vi "getRelPositions.vi"(9 "originOffsetVectors":T2, 10 "point":T1, 11 "mountOn":enum16{"yArm", "breadBoard"}(ring)) -> (2 "to_yPOI":T1, 3 "to_BBorigin":T1)   [LabVIEW 2015]
uses:
  <vilib>/Utility/miscctls.llb/LV3DPointTypeDef.ctl
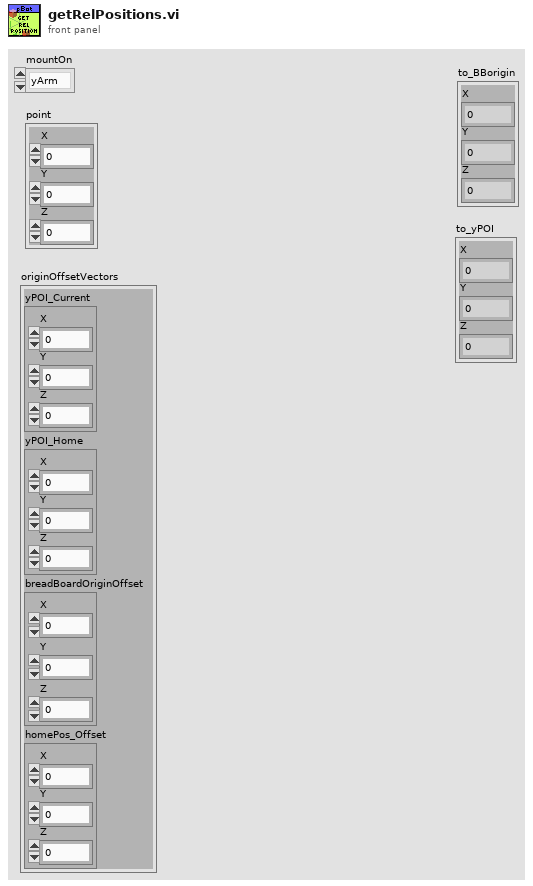
[diagram p1: front panel]
types:
  T1 = typedef "LV3DPointTypeDef.ctl" = cluster{"X":sgl, "Y":sgl, "Z":sgl}
  T2 = cluster{"yPOI_Current":T1, "yPOI_Home":T1, "breadBoardOriginOffset":cluster{"X":dbl, "Y":dbl, "Z":dbl}, "homePos_Offset":T1}
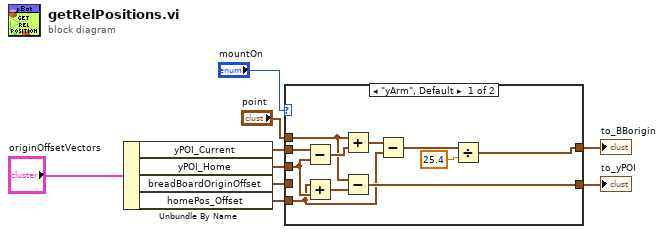
[diagram p0: block diagram]
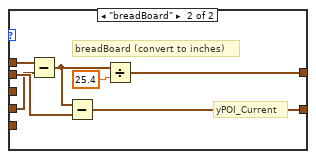
[diagram p2: hidden frame]
diagram:
  n1 = Unbundle By Name("originOffsetVectors") -> ("yPOI_Current"=w4:T1, "yPOI_Home"=w3:T1, "breadBoardOriginOffset"=w2:cluster{"X":dbl, "Y":dbl, "Z":dbl}, "homePos_Offset"=w1:T1)
  n2 = case shown="\"yArm\", Default" "mountOn" {
    tunnel: "point" -> [w12 w27]
    tunnel: w2 -> [_ w22]
    tunnel: w4 -> [w20 w26]
    tunnel: [w11 w21] -> w8
    tunnel: [w15 w24] -> w7
    tunnel: w3 -> [w14 _]
    tunnel: w1 -> [w10 _]
    frame "yArm", Default {
      n3 = Subtract(x=w20, y=w14) -> (x-y=w19:T1)
      n4 = Add(x=w10, y=w14) -> (x+y=w13:T1)
      n5 = Add(x=w12, y=w19) -> (x+y=w18:T1)
      n6 = Subtract(x=w12, y=w13) -> (x-y=w11:T1)
      n7 = Subtract(x=w18, y=w10) -> (x-y=w17:T1)
      n8 = Divide(x=w17, y=25.4) -> (x/y=w15:cluster{"X":dbl, "Y":dbl, "Z":dbl})
    }
    frame "breadBoard" {
      # "yPOI_Current"
      # "breadBoard (convert to inches)"
      n9 = Subtract(x=w27, y=w22) -> (x-y=w23:cluster{"X":dbl, "Y":dbl, "Z":dbl})
      n10 = Subtract(x=w23, y=w26) -> (x-y=w21:cluster{"X":dbl, "Y":dbl, "Z":dbl})
      n11 = Divide(x=w23, y=25.4) -> (x/y=w24:cluster{"X":dbl, "Y":dbl, "Z":dbl})
    }
  }
  "to_yPOI" <- w8
  "to_BBorigin" <- w7
